vi "Init.vi"(8 "error in (no error)":errorcluster, 11 "Execution Profiler In":refnum<class "Execution Profiler.lvclass">) -> (0 "error out":errorcluster, 3 "Execution Profiler Out":refnum<class "Execution Profiler.lvclass">)   [LabVIEW 2020, in "Execution Profiler.lvlib" / "Execution Profiler.lvclass"]
doc: "Initializes the process and creates necessary references. Anything initialized here is released in the Clear.vi method."
uses:
  Execution Profiler.lvclass
  Execution Profiler.lvclass/Execution Profiler.ctl
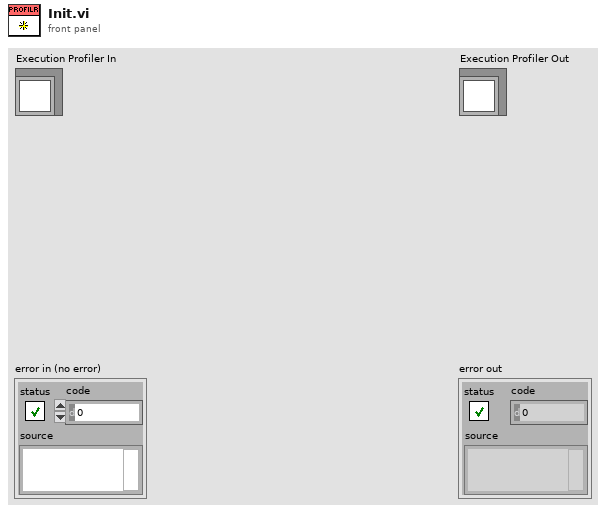
[diagram p1: front panel]
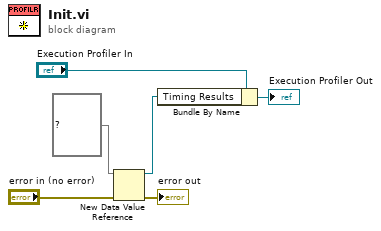
[diagram p0: block diagram]
diagram:
  n1 = New Data Value Reference(data value=map{string, dbl} {} ("Timing Results"), error in="error in (no error)") -> (data value reference=w1:refnum<data-value>, error out=→"error out":errorcluster)
  n2 = Bundle By Name(cluster="Execution Profiler In", "Timing Results"=w1) -> (→"Execution Profiler Out":refnum<class "Execution Profiler.lvclass">)
